vi "LTVUnicycleCtrl_Calculate.vi"(6 "RefAngularVelocity":dbl, 8 "RefLinearVelocity":dbl, 9 "RefPose":T2={"TRANSLATION"={"X"=0.0, "Y"=0.0}, "ROTATION"={"VALUE"=0.0, "COS"=1.0, "SIN"=0.0}} {"ROTATION"."SIN" format="%13.4f"; "ROTATION"."COS" format="%13.4f"; "ROTATION"."VALUE" format="%13.4f"; "TRANSLATION"."Y" format="%14.3f"; "TRANSLATION"."X" format="%14.3f"}, 10 "CurrentPose":T2={"TRANSLATION"={"X"=0.0, "Y"=0.0}, "ROTATION"={"VALUE"=0.0, "COS"=1.0, "SIN"=0.0}} {"ROTATION"."SIN" format="%13.4f"; "ROTATION"."COS" format="%13.4f"; "ROTATION"."VALUE" format="%13.4f"; "TRANSLATION"."Y" format="%14.3f"; "TRANSLATION"."X" format="%14.3f"}, 11 "in LTV_UNICYCLE_CONTROLLER":T5={"States"=0, "Inputs"=0, "PoseError"={"TRANSLATION"={"X"=0.0, "Y"=0.0}, "ROTATION"={"VALUE"=0.0, "COS"=1.0, "SIN"=0.0}}, "PoseTolerance"={"TRANSLATION"={"X"=0.0, "Y"=0.0}, "ROTATION"={"VALUE"=0.0, "COS"=1.0, "SIN"=0.0}}, "Dt"=0.02, "Enabled"=FALSE, "LQR_K_Table"={"Table Xs"=[], "Table Ys"=[], "MinX"=0.0, "MaxX"=0.0, "ItemCount"=0, "Rows"=0, "Columns"=0}} {"PoseTolerance"."ROTATION"."SIN" format="%13.4f"; "PoseTolerance"."ROTATION"."COS" format="%13.4f"; "PoseTolerance"."ROTATION"."VALUE" format="%13.4f"; "PoseTolerance"."TRANSLATION"."Y" format="%14.3f"; "PoseTolerance"."TRANSLATION"."X" format="%14.3f"; "PoseError"."ROTATION"."SIN" format="%13.4f"; "PoseError"."ROTATION"."COS" format="%13.4f"; "PoseError"."ROTATION"."VALUE" format="%13.4f"; "PoseError"."TRANSLATION"."Y" format="%14.3f"; "PoseError"."TRANSLATION"."X" format="%14.3f"}) -> (0 "Error":bool, 2 "ChassisSpeeds":T1 {"vOmega" format="%10.3f"; "vY" format="%10.3f"; "vX" format="%10.3f"}, 3 "out LTV_UNICYCLE_CONTROLLER":T5={"States"=0, "Inputs"=0, "PoseError"={"TRANSLATION"={"X"=0.0, "Y"=0.0}, "ROTATION"={"VALUE"=0.0, "COS"=1.0, "SIN"=0.0}}, "PoseTolerance"={"TRANSLATION"={"X"=0.0, "Y"=0.0}, "ROTATION"={"VALUE"=0.0, "COS"=1.0, "SIN"=0.0}}, "Dt"=0.02, "Enabled"=FALSE, "LQR_K_Table"={"Table Xs"=[], "Table Ys"=[], "MinX"=0.0, "MaxX"=0.0, "ItemCount"=0, "Rows"=0, "Columns"=0}} {"PoseTolerance"."ROTATION"."SIN" format="%13.4f"; "PoseTolerance"."ROTATION"."COS" format="%13.4f"; "PoseTolerance"."ROTATION"."VALUE" format="%13.4f"; "PoseTolerance"."TRANSLATION"."Y" format="%14.3f"; "PoseTolerance"."TRANSLATION"."X" format="%14.3f"; "PoseError"."ROTATION"."SIN" format="%13.4f"; "PoseError"."ROTATION"."COS" format="%13.4f"; "PoseError"."ROTATION"."VALUE" format="%13.4f"; "PoseError"."TRANSLATION"."Y" format="%14.3f"; "PoseError"."TRANSLATION"."X" format="%14.3f"})   [LabVIEW 2019, in "Trajectory_Library.lvlib"]
doc: "Returns the linear and angular velocity outputs of the LTV controller.\n\nInputs:\n - in LTV Unicycle Controller -- Controller data cluster\n - currentPose -- The current pose.\n - poseRef -- The desired pose. (Setpont)\n - linearVelocityRef -- The desired linear velocity in meters per second. (Feedforward)\n - angularVelocityRef -- The desired angular velocity in radians per second. (Feedforward)\n\nOutputs:\n - out LTV Unicycle Controller -- Updatated data cluster\n - Chassis Speeds -- The linear and angular velocity outputs of the LTV controller.\n - Error -- Returns TRUE if an error occured."
uses:
  Trajectory_Library.lvlib
  <vilib>/Analysis/NI_AALBase.lvlib
  <vilib>/Analysis/baseanly.llb/Real A x B.vi
  TypeDef/LTV_UNICYCLE_CONTROLLER.ctl
  TypeDef/TRANSLATION2D.ctl
  TypeDef/ROTATION2D.ctl
  TypeDef/POSE2D.ctl
  TypeDef/CHASSIS_SPEEDS.ctl
  TypeDef/FUNCTION_GENERATOR_MATRIX.ctl
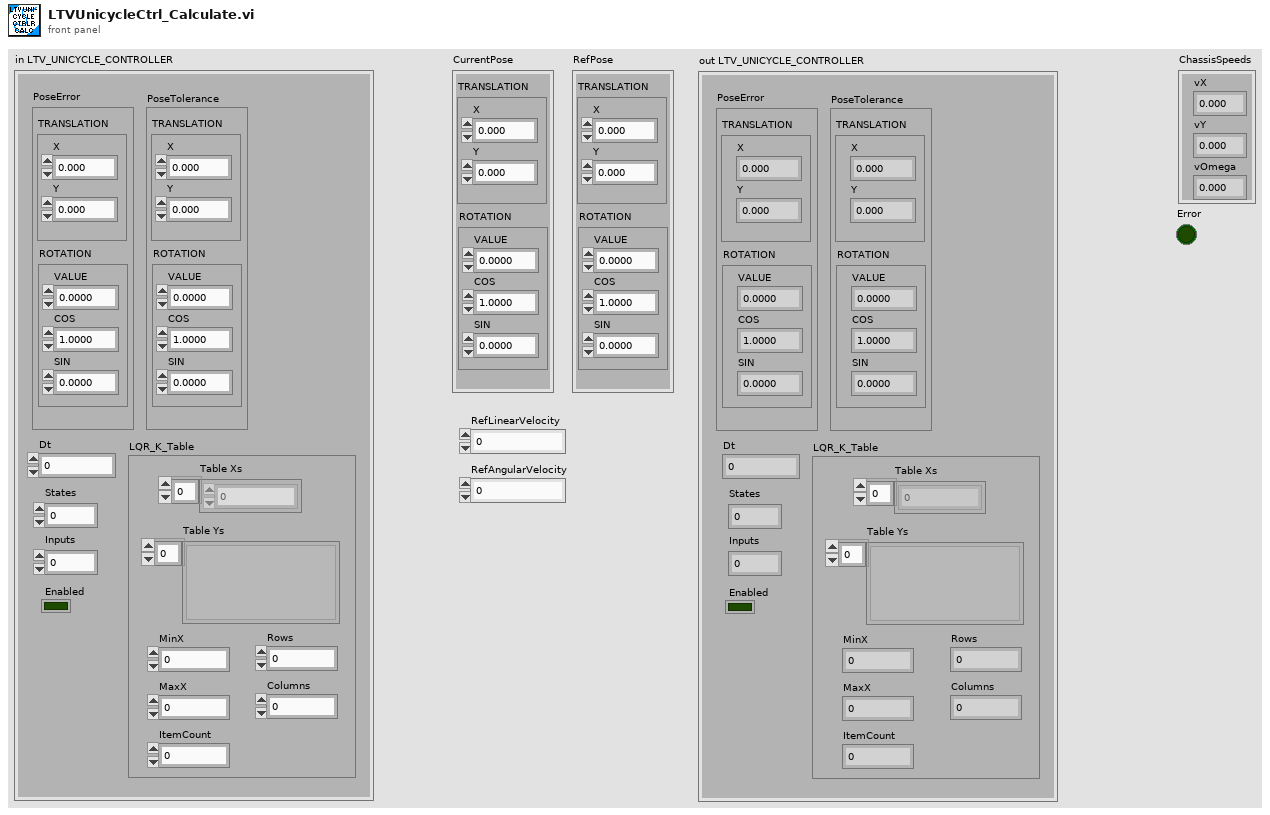
[diagram p1: front panel]
types:
  T1 = typedef "Trajectory_Library.lvlib/CHASSIS_SPEEDS.ctl" = cluster{"vX":dbl, "vY":dbl, "vOmega":dbl}
  T2 = typedef "Trajectory_Library.lvlib/POSE2D.ctl" = cluster{"TRANSLATION":T3, "ROTATION":T4}
  T3 = typedef "Trajectory_Library.lvlib/TRANSLATION2D.ctl" = cluster{"X":dbl, "Y":dbl}
  T4 = typedef "Trajectory_Library.lvlib/ROTATION2D.ctl" = cluster{"VALUE":dbl, "COS":dbl, "SIN":dbl}
  T5 = typedef "Trajectory_Library.lvlib/LTV_UNICYCLE_CONTROLLER.ctl" = cluster{"States":i32, "Inputs":i32, "PoseError":T2, "PoseTolerance":T2, "Dt":dbl, "Enabled":bool, "LQR_K_Table":T6}
  T6 = typedef "Trajectory_Library.lvlib/FUNCTION_GENERATOR_MATRIX.ctl" = cluster{"Table Xs":dbl[], "Table Ys":variant[], "MinX":dbl, "MaxX":dbl, "ItemCount":i32, "Rows":i32, "Columns":i32}
  T7 = typedef "NI_Matrix.lvlib/RealMatrix.ctl" = dbl[][]
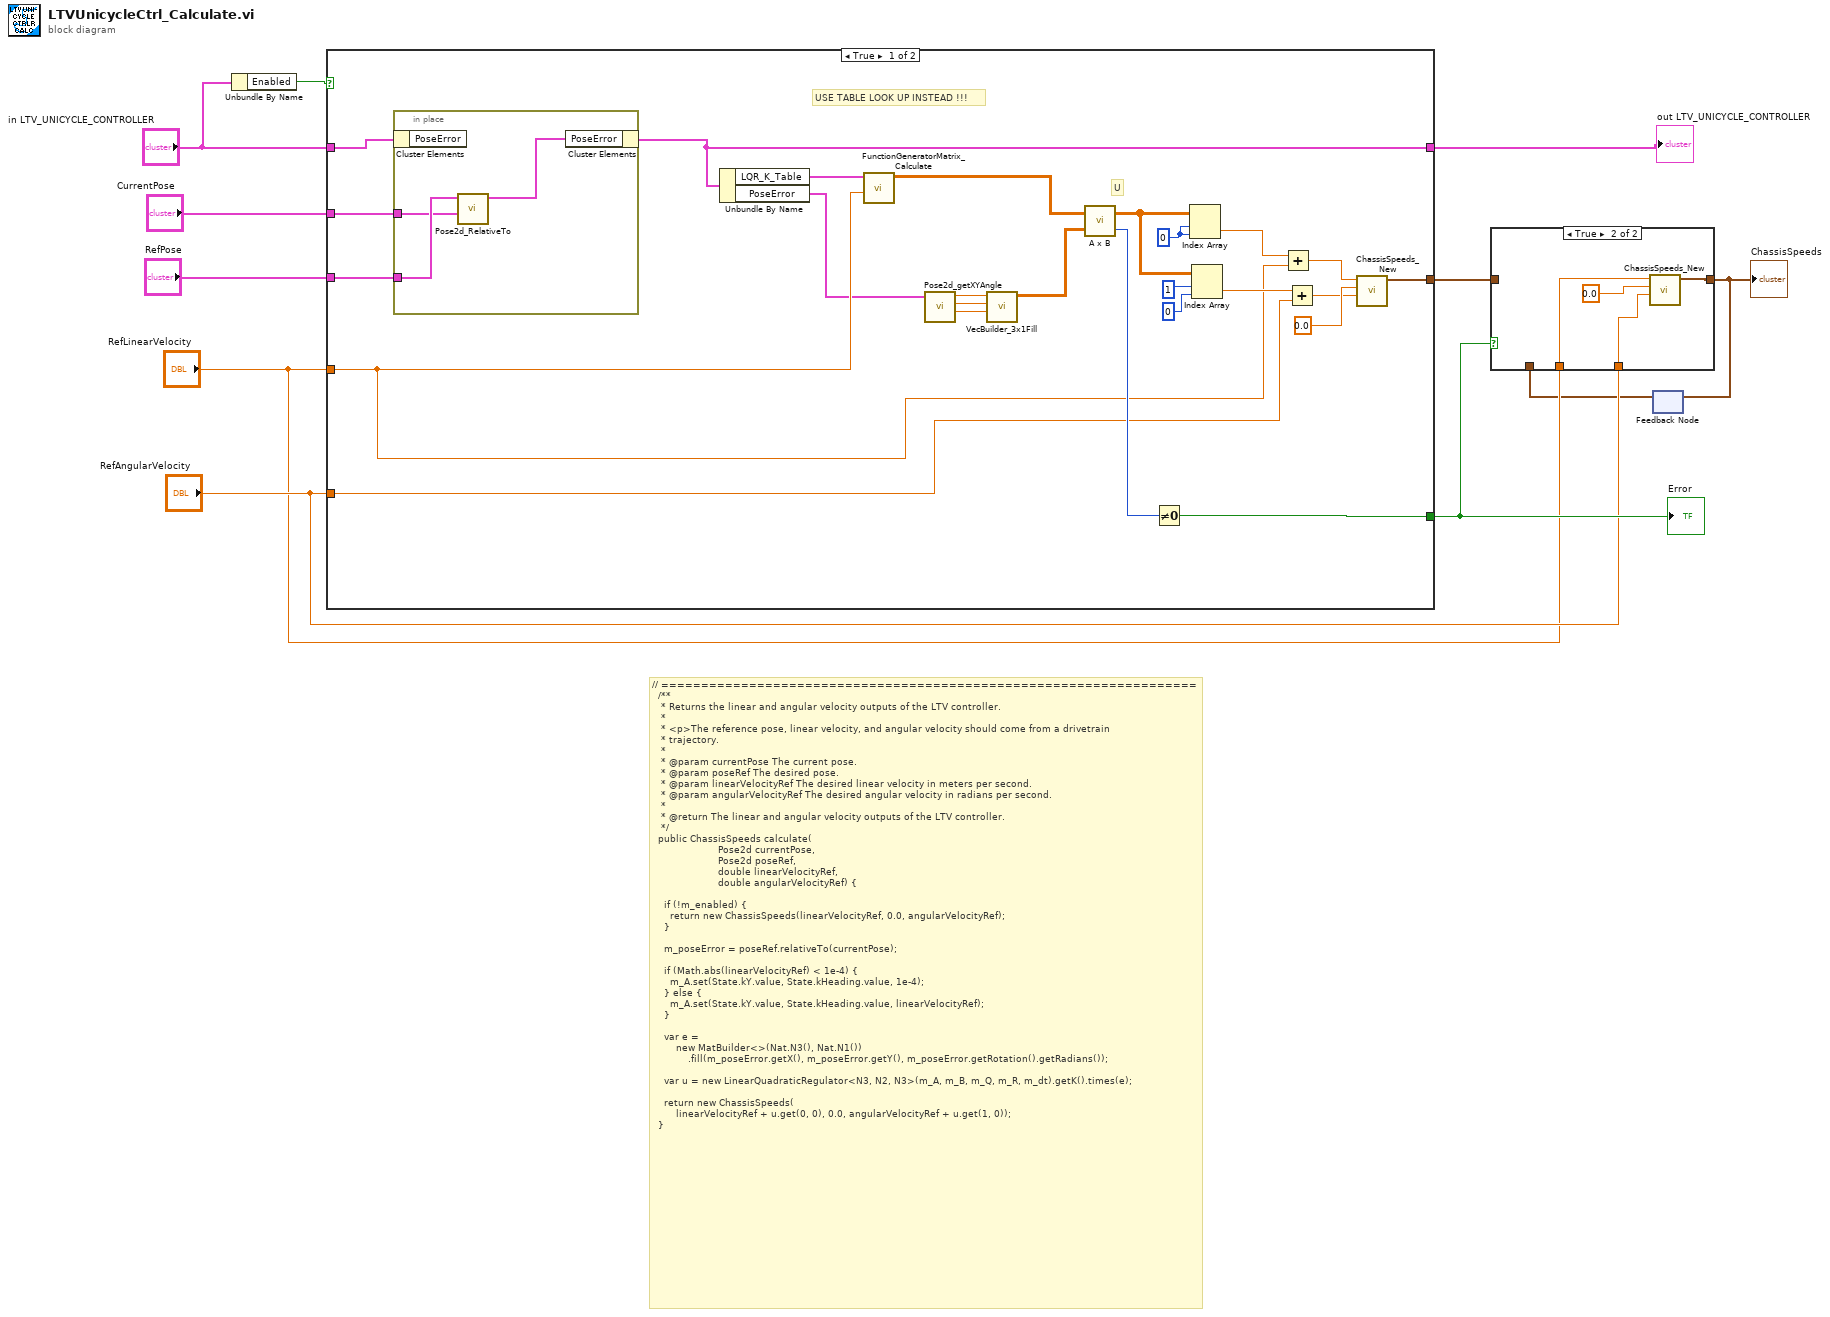
[diagram p0: block diagram]
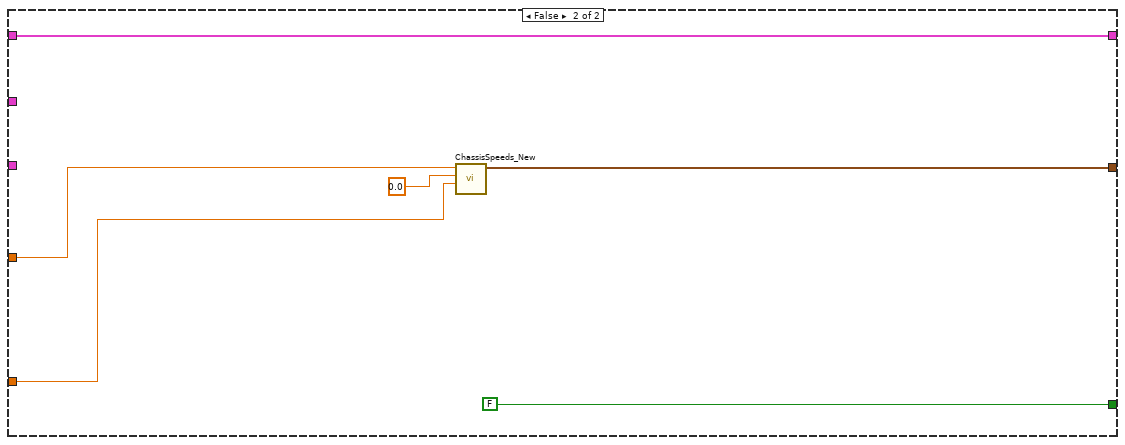
[diagram p3: hidden frame]
diagram:
  # "// ===================================================================\n  /**\n   * Returns the linear and angular velocity outputs of the LTV controller.\n   *\n   * <p>The reference pose, linear velocity, and angular velocity should come from a drivetrain\n   * trajectory.\n   *\n   * @param currentPose The current pose.\n   * @param poseRef The desired pose.\n   * @param linearVelocityRef The desired linear velocity in meters per second.\n   * @param angularVelocityRef The desired angular velocity in radians per second.\n   *\n   * @return The linear and angular velocity outputs of the LTV controller.\n   */\n  public ChassisSpeeds calculate(\n      \t               Pose2d currentPose, \n       \t              Pose2d poseRef, \n\t                     double linearVelocityRef, \n\t                     double angularVelocityRef) {\n\n    if (!m_enabled) {\n      return new ChassisSpeeds(linearVelocityRef, 0.0, angularVelocityRef);\n    }\n\n    m_poseError = poseRef.relativeTo(currentPose);\n\n    if (Math.abs(linearVelocityRef) < 1e-4) {\n      m_A.set(State.kY.value, State.kHeading.value, 1e-4);\n    } else {\n      m_A.set(State.kY.value, State.kHeading.value, linearVelocityRef);\n    }\n\n    var e =\n        new MatBuilder<>(Nat.N3(), Nat.N1())\n            .fill(m_poseError.getX(), m_poseError.getY(), m_poseError.getRotation().getRadians());\n\n    var u = new LinearQuadraticRegulator<N3, N2, N3>(m_A, m_B, m_Q, m_R, m_dt).getK().times(e);\n\n    return new ChassisSpeeds(\n        linearVelocityRef + u.get(0, 0), 0.0, angularVelocityRef + u.get(1, 0));\n  }"
  n1 = Unbundle By Name("in LTV_UNICYCLE_CONTROLLER") -> ("Enabled"=w11:bool)
  n2 = case shown="True" w11 {
    tunnel: "in LTV_UNICYCLE_CONTROLLER" -> [w36 w45]
    tunnel: [w33 w45] -> w9
    tunnel: [w12 FALSE] -> w6
    tunnel: [w27 w43] -> w5
    tunnel: "RefLinearVelocity" -> [w15 w42]
    tunnel: "RefAngularVelocity" -> [w23 w41]
    tunnel: "RefPose" -> [w35 _]
    tunnel: "CurrentPose" -> [w34 _]
    frame True {
      w22 = 0 ("index (row)")
      # "U"
      # "USE TABLE LOOK UP INSTEAD !!!"
      n3 = in-place {
        in-place-border: w35 -> [w39]
        in-place-border: w34 -> [w38]
        n4 = in-place-cluster #1(w36) -> ()  [unwired: 1 out]
        n5 = call "Pose2d_RelativeTo.vi"("other POSE"=w38, "in POSE"=w39) -> ("out POSE"=w37:T2)  [unwired: 9 in]
        n6 = in-place-cluster #1("PoseError"=w37) -> (w33:T5)
      }
      n7 = Unbundle By Name(w33) -> ("LQR_K_Table"=w16:T6, "PoseError"=w14:T2)
      n8 = call "FunctionGeneratorMatrix_Calculate.vi"("Input Value"=w15, "FUNCTION_GENERATOR_MATRIX"=w16) -> ("Output Matrix"=w13:T7)  [unwired: 9 in]
      n9 = call "Pose2d_getXYAngle.vi"("in POSE"=w14) -> ("Angle"=w30:dbl, "Y"=w31:dbl, "X"=w32:dbl)  [unwired: 8 in]
      n10 = call "VecBuilder_3x1Fill.vi"("R2"=w30, "R1"=w31, "R0"=w32) -> ("output matrix"=w29:T7)  [unwired: 8 in]
      n11 = call-poly <vilib>:"A x B.vi"("B"=w29, "A"=w13) -> ("error"=w28:i32, "A x B"=w19:T7)
      n12 = Not Equal To 0?(x=w28) -> (x != 0?=w12:bool)
      n13 = Index Array(array=w19, index (row)=w22, index (col)=w22) -> (element=w18:dbl)
      n14 = Index Array(array=w19, index (row)=1, index (col)=0 ("index (row)")) -> (element=w17:dbl)
      n15 = Add(x=w18, y=w15) -> (x+y=w25:dbl)
      n16 = Add(x=w17, y=w23) -> (x+y=w24:dbl)
      n17 = call "ChassisSpeeds_New.vi"("vAngular"=w24, "vY"=0.0, "vX"=w25) -> ("CHASSIS"=w27:T1)  [unwired: 8 in]
    }
    frame False {
      n18 = call "ChassisSpeeds_New.vi"("vAngular"=w41, "vY"=0.0, "vX"=w42) -> ("CHASSIS"=w43:T1)  [unwired: 8 in]
    }
  }
  "out LTV_UNICYCLE_CONTROLLER" <- w9
  "Error" <- w6
  n19 = feedback #2() -> (w1:T1)  [unwired: 1 in]
  n20 = case shown="True" w6 {
    tunnel: w5 -> [w46 _]
    tunnel: [w46 w47] -> w2
    tunnel: "RefAngularVelocity" -> [_ w49]
    tunnel: "RefLinearVelocity" -> [_ w48]
    tunnel: w1 -> [_ _]
    frame False {
    }
    frame True {
      n21 = call "ChassisSpeeds_New.vi"("vAngular"=w49, "vY"=0.0, "vX"=w48) -> ("CHASSIS"=w47:T1)  [unwired: 8 in]
    }
  }
  "ChassisSpeeds" <- w2
  n22 = feedback-in #2(w2) -> ()
